vi "decode string.vi"(11 "byte array in":u8[](array[numeric]) format="%.0b") -> (3 "String":string)   [LabVIEW 2013, in "protocol buffers encoder.lvlib"]
uses:
  protocol buffers encoder.lvlib
panel:
  out "mgerr":i32
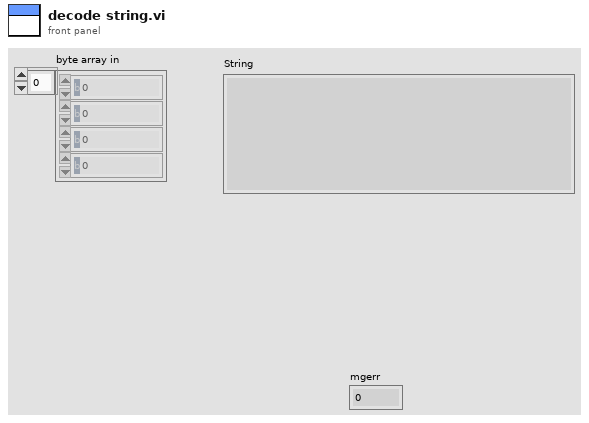
[diagram p1: front panel]
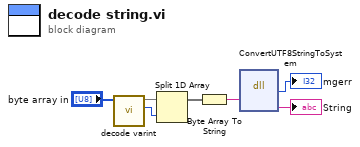
[diagram p0: block diagram]
diagram:
  n1 = call "decode varint.vi"("byte array in"="byte array in") -> ("read index out"=w5:i32, 3:w6)  [unwired: 8 in, 1 out]
  n2 = Split 1D Array(array=w6, index=w5) -> (first subarray=w4:void[])  [unwired: 1 out]
  n3 = Byte Array To String(unsigned byte array=w4) -> (string=w1:string)
  n4 = dll-call lib="LabVIEW" fn="ConvertUTF8StringToSystem"("input"=w1) -> ("mgerr"=→"mgerr":i32, "output"=→"String":string)  [unwired: 5 in, 2 out]
